vi "updateAutoExposure.vi"(8 "error in (no error)":errorcluster, 10 "force":bool, 11 "Camera in":refnum<class "Camera.lvclass">) -> (0 "error out":errorcluster, 3 "Camera out":refnum<class "Camera.lvclass">)   [LabVIEW 2019, in "Camera.lvclass"]
doc: "Make changes to the settings of the auto-exposure mode"
uses:
  Camera.lvclass
  Camera.lvclass/Camera.ctl
  pco.recorder/Recorder.lvlib
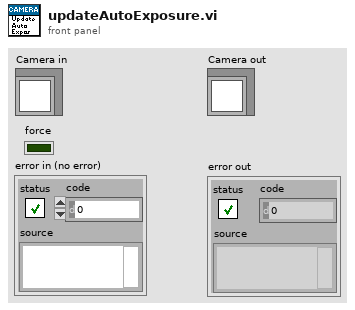
[diagram p1: front panel]
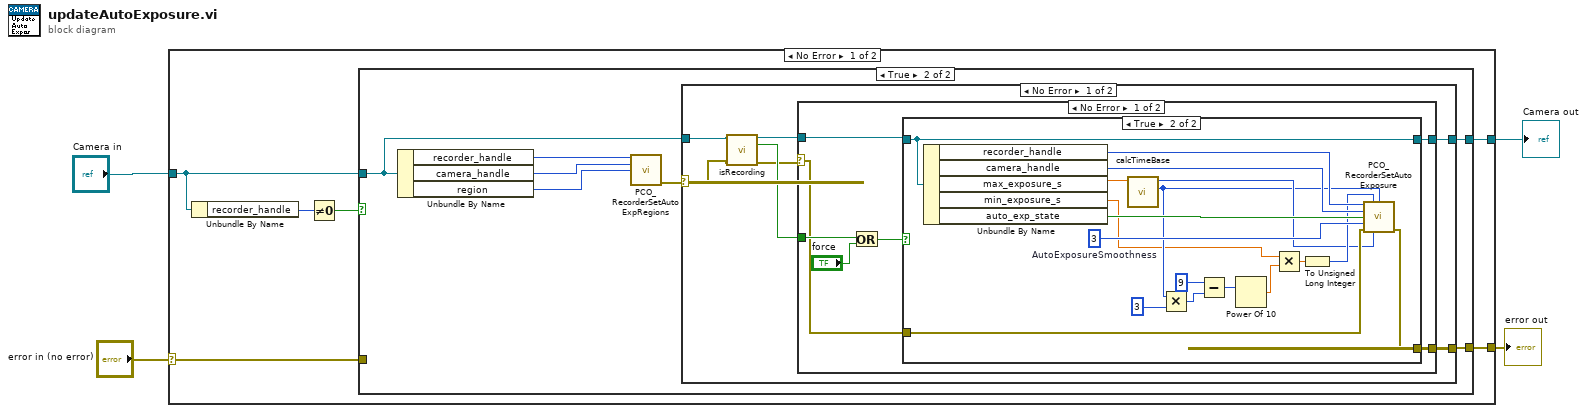
[diagram p0: block diagram]
diagram:
  n1 = case shown="No Error" "error in (no error)" {
    selector: "error in (no error)" -> [w8 w58]
    tunnel: "Camera in" -> [w7 w59]
    tunnel: [w10 w59] -> w2
    tunnel: [w9 w58] -> w1
    frame No Error {
      n2 = Unbundle By Name(w7) -> ("recorder_handle"=w6:u64)
      n3 = Not Equal To 0?(x=w6) -> (x != 0?=w5:bool)
      n4 = case shown="True" w5 {
        tunnel: [w12 w13] -> w10
        tunnel: [w11 w15] -> w9
        tunnel: w8 -> [w11 _]
        tunnel: w7 -> [w12 w14]
        frame False {
        }
        frame True {
          n5 = Unbundle By Name(w14) -> ("recorder_handle"=w19:u64, "camera_handle"=w18:u64, "region"=w17:u16)
          n6 = call "PCO_RecorderSetAutoExpRegions.vi"("phRec"=w19, "phCam"=w18, "wRegionType"=w17) -> ("error out"=w16:errorcluster)  [unwired: 10 in, 2 out]
          n7 = case shown="No Error" w16 {
            selector: w16 -> [w24 w57]
            tunnel: [w22 w57] -> w15
            tunnel: w14 -> [w26 w56]
            tunnel: [w20 w56] -> w13
            frame No Error {
              n8 = call-dynamic "isRecording.vi"("Camera in"=w26, "error in (no error)"=w24) -> ("Camera out"=w21:refnum<class "Camera.lvclass">, "recording"=w25:bool, "error out"=w23:errorcluster)  [unwired: 11 in]
              n9 = case shown="No Error" w23 {
                selector: w23 -> [w28 w55]
                tunnel: w25 -> [w33 _]
                tunnel: [w27 w55] -> w22
                tunnel: w21 -> [w30 w54]
                tunnel: [w29 w54] -> w20
                frame No Error {
                  n10 = Or(x=w33, y="force") -> (x .or. y?=w31:bool)
                  n11 = case shown="True" w31 {
                    tunnel: w30 -> [w35 w53]
                    tunnel: [w35 w53] -> w29
                    tunnel: w28 -> [w34 w49]
                    tunnel: [w34 w48] -> w27
                    frame False {
                    }
                    frame True {
                      w46 = u16 3  # AutoExposureSmoothness
                      n12 = Unbundle By Name(w53) -> ("recorder_handle"=w51:u64, "camera_handle"=w50:u64, "max_exposure_s"=w52:dbl, "min_exposure_s"=w36:dbl, "auto_exp_state"=w47:bool)
                      n13 = call "calcTimeBase.vi"("time"=w52) -> ("base_calculated"=w37:u16, "time_calculated"=w38:u32)  [unwired: 9 in]
                      n14 = Multiply(x=w37, y=3) -> (x*y=w44:i32)
                      n15 = Subtract(x=9, y=w44) -> (x-y=w42:i32)
                      n16 = Power Of 10(x=w42) -> (10^x=w41:dbl)
                      n17 = Multiply(x=w36, y=w41) -> (x*y=w40:dbl)
                      n18 = To Unsigned Long Integer(number=w40) -> (unsigned 32bit integer=w39:u32)
                      n19 = call "PCO_RecorderSetAutoExposure.vi"("phRec"=w51, "dwMinExposure"=w39, "wExpBase"=w37, "phCam"=w50, "bAutoExpState"=w47, "wSmoothness"=w46, "error in (no error)"=w49, "dwMaxExposure"=w38) -> ("error out"=w48:errorcluster)  [unwired: 5 in, 2 out]
                    }
                  }
                }
                frame Error {
                }
              }
            }
            frame Error {
            }
          }
        }
      }
    }
    frame Error {
    }
  }
  "Camera out" <- w2
  "error out" <- w1
